vi "Not An SFTP Refnum.vi"(1 "sftp":T1) -> (0 "Not a SFTP Refnum?":bool)   [LabVIEW 2017, in "libssh2.lvlib"]
doc: "Returns TRUE if <B>sftp</B> is not an SFTP refnum. Otherwise, FALSE."
uses:
  libssh2.lvlib
  SFTP Refnum.ctl
  SFTP Refnum Data.ctl
  Session Refnum.ctl
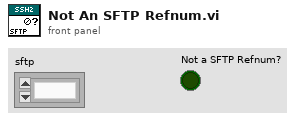
[diagram p1: front panel]
types:
  T1 = typedef "libssh2.lvlib/SFTP Refnum.ctl" = refnum<k1>
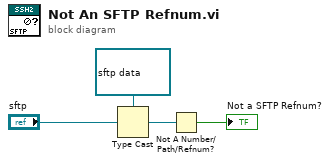
[diagram p0: block diagram]
diagram:
  n1 = Type Cast(type=refnum<data-value> refnum ("data value reference"), x="sftp") -> (*(type *) &x=w2:refnum<data-value>)
  n2 = Not A Number/Path/Refnum?(number/path/refnum=w2) -> (NaN/Path/Refnum?=→"Not a SFTP Refnum?":bool)
